vi "fgv_PXI-5110.vi"(7 "cmd":T1(ring), 8 "error in":errorcluster) -> (0 "error out":errorcluster)   [LabVIEW 2021]
uses:
  ctrl/ini-rw.ctl
  ctrl/5110_q.ctl
  <instrlib>/niScope/Utility/niScope Get Channel Name From String.vi
  <instrlib>/niScope/Configure/Trigger/niScope Configure Trigger Edge.vi
  <instrlib>/niScope/Acquire/Fetch/niScope Multi Fetch Cluster.vi
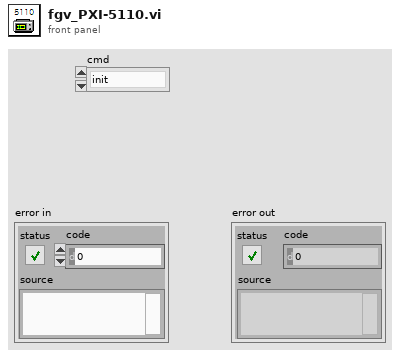
[diagram p1: front panel]
types:
  T1 = enum16{"init", "config", "trigger", "read", "close"}
  T2 = typedef "ini-rw.ctl" = enum16{"read", "write", "ini"}
  T3 = typedef "5110_q.ctl" = enum16{"create", "read", "write", "close"}
  T4 = cluster{"Waveform(s)":cluster{"relativeInitialX":dbl, "xIncrement":dbl, "wfm":dbl[]}[], "Actual Record Length":i32, "Actual Sample Rate":dbl, "Auto Triggered":bool}
  T5 = typedef "5110_trigger.ctl" = cluster{"visa":refnum<k15>, "Channel Name":string, "Enforce Realtime":bool, "Vertical Range":dbl, "Min Sample Rate":dbl, "Min Record Length":i32, "Actual Record Length":i32, "Actual Sample Rate":dbl, "Timeout (s)":dbl, "Vertical Offset":dbl, "Probe Attenuation":dbl, "Input Impedance":u32, "Maximum Input Frequency":dbl, "Vertical Coupling":i32, "Trigger":cluster{"Coupling":u16, "Trigger Slope":i32, "Trigger Level":dbl, "Trigger Source":string, "Trigger Delay":dbl, "Reference Position":dbl, "Trigger Modifier":i32, "Auto Triggered":bool}}
  T6 = cluster{"relativeInitialX":dbl, "xIncrement":dbl, "wfm":dbl[]}[]
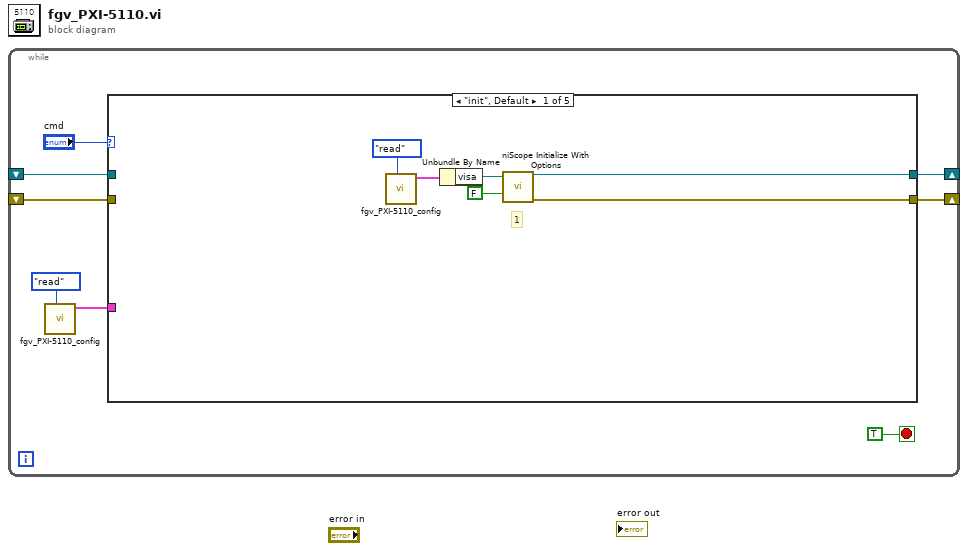
[diagram p0: block diagram]
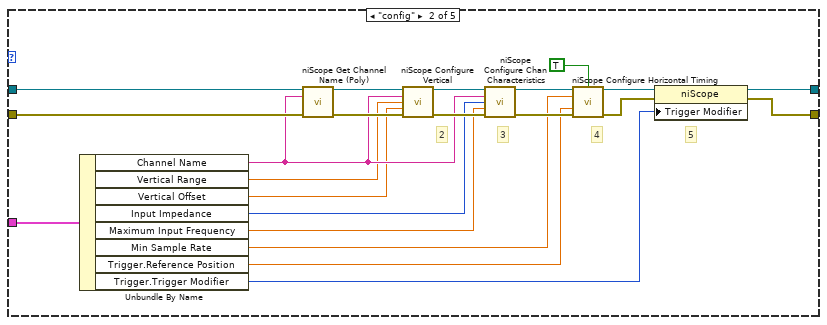
[diagram p2: hidden frame]
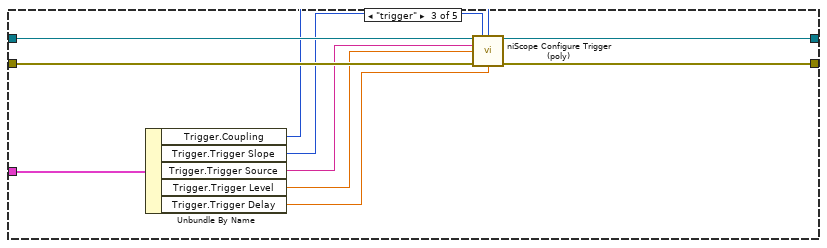
[diagram p3: hidden frame]
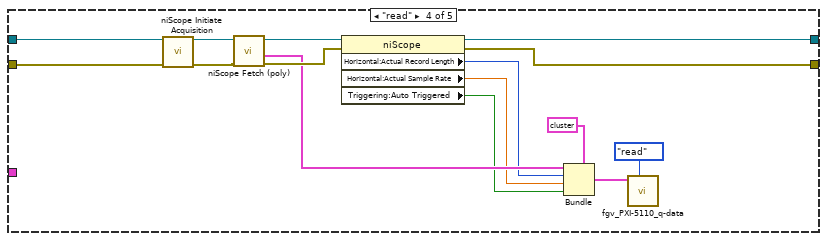
[diagram p4: hidden frame]
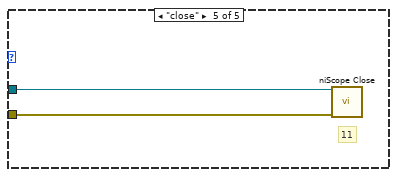
[diagram p5: hidden frame]
diagram:
  n1 = while {
    shift-right: [w6] -> _
    shift-left: _ -> [w4]
    shift-right: [w5] -> _
    shift-left: _ -> [w3]
    stop <- TRUE stop-if-true
    n2 = call "fgv_PXI-5110_config.vi"("cmd"=ini-rw."read") -> ("cfg 2"=w2:T5)  [unwired: 10 in]
    n3 = case shown="\"init\", Default" "cmd" {
      tunnel: [w13 w24 w46 w55 _] -> w6
      tunnel: [w12 w25 w45 w54 _] -> w5
      tunnel: w4 -> [_ w27 w44 w57 w63]
      tunnel: w3 -> [_ w26 w43 w56 w62]
      tunnel: w2 -> [_ w15 w37 _ _]
      frame "init", Default {
        # "1"
        n4 = call "fgv_PXI-5110_config.vi"("cmd"=ini-rw."read") -> ("cfg 2"=w10:T5)  [unwired: 10 in]
        n5 = Unbundle By Name(w10) -> ("visa"=w9:refnum<k15>)
        n6 = call <instrlib>:"niScope Initialize With Options.vi"("resource name"=w9, "reset device"=FALSE ("Reset Device")) -> ("instrument handle"=w13:refnum<k15>, "error out"=w12:errorcluster)  [unwired: 12 in]
      }
      frame "config" {
        # "5"
        # "2"
        # "3"
        # "4"
        n7 = Unbundle By Name(w15) -> ("Channel Name"=w23:string, "Vertical Range"=w22:dbl, "Vertical Offset"=w21:dbl, "Input Impedance"=w20:u32, "Maximum Input Frequency"=w19:dbl, "Min Sample Rate"=w18:dbl, "Trigger.Reference Position"=w17:dbl, "Trigger.Trigger Modifier"=w16:i32)
        n8 = call-poly <instrlib>:"niScope Get Channel Name (Poly).vi"("instrument handle"=w27, "index"=w23, "error in"=w26) -> ("instrument handle out"=w29:refnum<k15>, "error out"=w28:errorcluster)  [unwired: 10 in, 1 out]
        n9 = call <instrlib>:"niScope Configure Vertical.vi"("instrument handle"=w29, "channels"=w23, "vertical range"=w22, "vertical offset"=w21, "error in"=w28) -> ("instrument handle out"=w36:refnum<k15>, "error out"=w35:errorcluster)  [unwired: 9 in]
        n10 = call <instrlib>:"niScope Configure Chan Characteristics.vi"("instrument handle"=w36, "channels"=w23, "input impedance"=w20, "maximum input frequency"=w19, "error in"=w35) -> ("instrument handle out"=w33:refnum<k15>, "error out"=w34:errorcluster)  [unwired: 9 in]
        n11 = call <instrlib>:"niScope Configure Horizontal Timing.vi"("instrument handle"=w33, "enforce realtime"=TRUE ("Enforce Realtime"), "min sample rate"=w18, "reference position"=w17, "error in"=w34) -> ("instrument handle out"=w32:refnum<k15>, "error out"=w31:errorcluster)  [unwired: 9 in]
        n12 = property on="Property Node" class="niScope"(reference=w32, error in=w31, "Trigger Modifier"=w16) -> (reference out=w24:refnum<k15>, error out=w25:errorcluster)
      }
      frame "trigger" {
        n13 = Unbundle By Name(w37) -> ("Trigger.Coupling"=w42:u16, "Trigger.Trigger Slope"=w41:i32, "Trigger.Trigger Source"=w40:string, "Trigger.Trigger Level"=w39:dbl, "Trigger.Trigger Delay"=w38:dbl)
        n14 = call-poly <instrlib>:"niScope Configure Trigger (poly).vi"("instrument handle"=w44, "trigger slope"=w41, "trigger coupling"=w42, "trigger source"=w40, "trigger level"=w39, "error in"=w43, "trigger delay"=w38) -> ("instrument handle out"=w46:refnum<k15>, "error out"=w45:errorcluster)  [unwired: 7 in]
      }
      frame "read" {
        n15 = call <instrlib>:"niScope Initiate Acquisition.vi"("instrument handle"=w57, "error in"=w56) -> ("instrument handle out"=w61:refnum<k15>, "error out"=w60:errorcluster)  [unwired: 12 in]
        n16 = call-poly <instrlib>:"niScope Fetch (poly).vi"("error in"=w60, "instrument handle"=w61) -> ("error out"=w58:errorcluster, "waveform"=w52:T6, "instrument handle out"=w59:refnum<k15>)  [unwired: 6 in, 1 out]
        n17 = property class="niScope"(reference=w59, error in=w58) -> (reference out=w55:refnum<k15>, error out=w54:errorcluster, "Horizontal:Actual Record Length"=w51:i32, "Horizontal:Actual Sample Rate"=w50:dbl, "Triggering:Auto Triggered"=w49:bool)
        n18 = Bundle(cluster=T4 {"Waveform(s)"=[{"relativeInitialX"=-2.0906779296874975e-05, "xIncrement"=1e-07, "wfm"=array[3000 elements]}], "Actual Record Length"=3000, "Actual Sample Rate"=10000000.0, "Auto Triggered"=FALSE} ("data 2"), "Waveform(s)"=w52, "Actual Record Length"=w51, "Actual Sample Rate"=w50, "Auto Triggered"=w49) -> (w47:T4)
        n19 = call "fgv_PXI-5110_q-data.vi"("cmd"=5110_q."read", "data 2"=w47) -> ()  [unwired: 8 in, 2 out]
      }
      frame "close" {
        # "11"
        n20 = call <instrlib>:"niScope Close.vi"("instrument handle"=w63, "error in"=w62) -> ()  [unwired: 13 in, 1 out]
      }
    }
  }
